vi "Untitled 4.vi"() -> ()   [LabVIEW 2013]
uses:
  <vilib>/rvi/Emulation/niFpgaSctlEmulationGetInTimedLoop.vi
  <vilib>/rvi/Emulation/niFpgaEmulationReportErrorSimple.vi
  <vilib>/rvi/Emulation/niFpgaGetClockAttributes.vi
  <vilib>/rvi/eio/common/nirviEmuTemplateMethod_errors.vi
  <vilib>/rvi/Emulation/niFpgaCriticalErrorInLSC.vi
  <vilib>/eio/EIONode/EIONode.xnode
panel:
  out "x-y":u32
  out "s? t:f":fxp<+/-,32,16>
  in  "reset":bool
  out "Z":bool
  out "B":bool
  out "A":bool
  in  "stop":bool
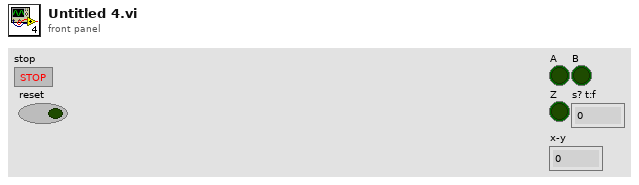
[diagram p1: front panel]
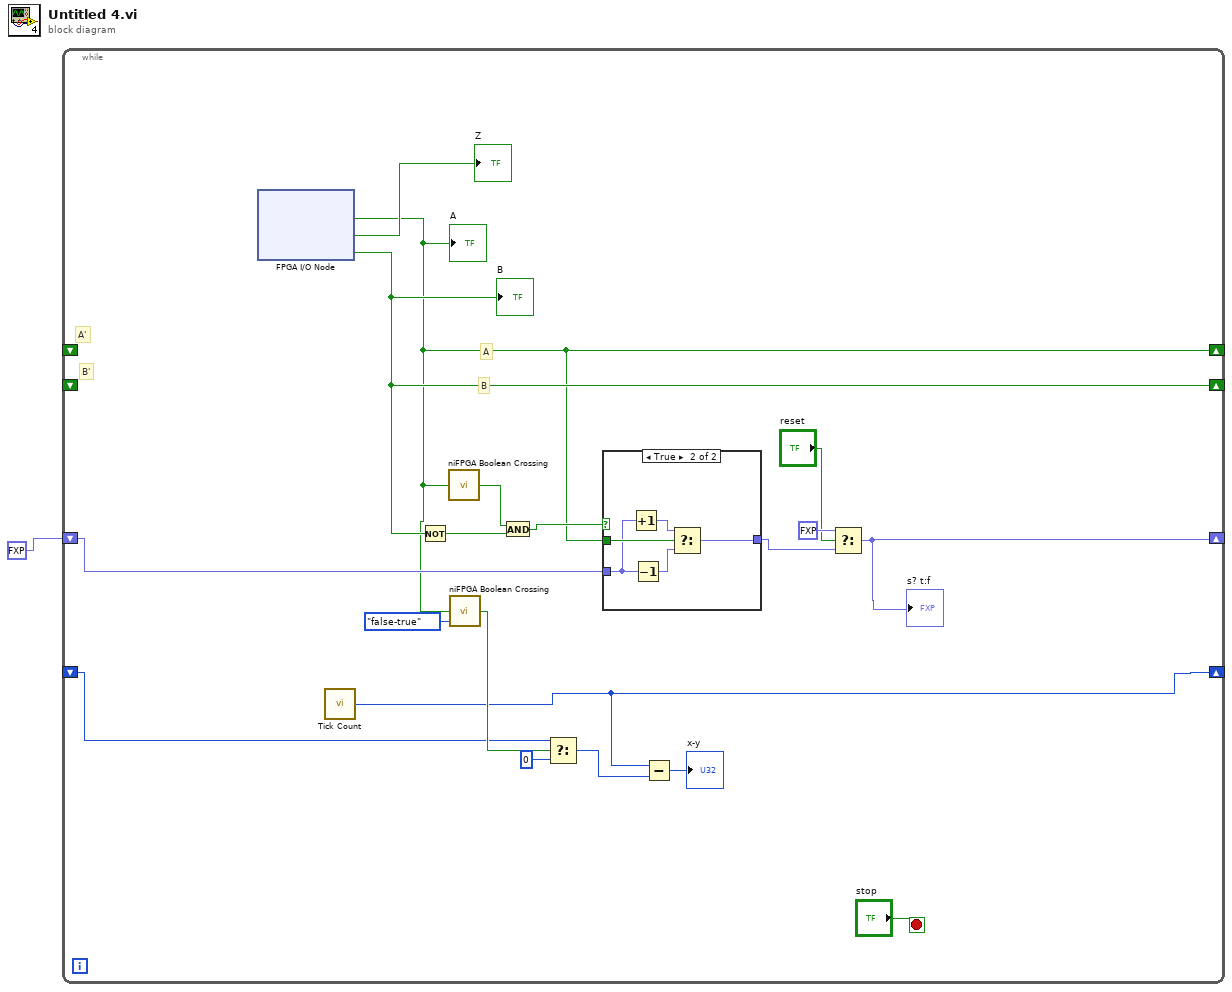
[diagram p0: block diagram]
diagram:
  n1 = while {
    shift-right: [w9] -> _
    shift-left: _ -> [_]
    shift-right: [w16] -> _
    shift-left: _ -> [_]
    shift-right: [w10] -> _
    shift-left: fxp<+,1,1> 0.0 -> [w13]
    shift-right: [w5] -> _
    shift-left: _ -> [w6]
    stop <- "stop" stop-if-true
    # "B'"
    # "A'"
    # "B"
    # "A"
    n2 = xnode "FPGA I/O Node"() -> ("Mod1/DI0"=w9:bool, "Mod1/DI1"=→"Z":bool, "Mod1/DI2"=w16:bool)  [unwired: 3 in, 3 out]
    "A" <- w9
    "B" <- w16
    n3 = call "Tick Count"() -> ("Tick Count(uSec)"=w5:u32)
    n4 = Not(x=w16) -> (.not. x?=w17:bool)
    n5 = call <vilib>:"niFPGA Boolean Crossing.vi"("input"=w9) -> ("crossing"=w11:bool)  [unwired: 8 in]
    n6 = call <vilib>:"niFPGA Boolean Crossing.vi"("input"=w9, "direction"=enum8{"either", "false-true", "true-false"}."false-true") -> ("crossing"=w7:bool)  [unwired: 7 in]
    n7 = And(x=w11, y=w17) -> (x .and. y?=w18:bool)
    n8 = Select(t=w6, s=w7, f=u32 0) -> (s? t:f=w4:u32)
    n9 = case shown="True" w18 {
      tunnel: w9 -> [_ w24]
      tunnel: [w21 w23] -> w15
      tunnel: w13 -> [w21 w22]
      frame False {
      }
      frame True {
        n10 = Increment(x=w22) -> (x+1=w25:fxp<+/-,32,16>)
        n11 = Decrement(x=w22) -> (x-1=w26:fxp<+/-,32,16>)
        n12 = Select(t=w25, s=w24, f=w26) -> (s? t:f=w23:fxp<+/-,32,16>)
      }
    }
    n13 = Subtract(x=w5, y=w4) -> (x-y=→"x-y":u32)
    n14 = Select(t=fxp<+,1,1> 0.0, s="reset", f=w15) -> (s? t:f=w10:fxp<+/-,32,16>)
    "s? t:f" <- w10
  }
